vi "SteeringControl.vi"(0 "Position (Counts)":i32, 1 "Roll rate (rad/s)":dbl, 2 "RollRef":dbl, 3 "Limit":i8, 4 "P gain":dbl, 5 "I gain":dbl, 6 "error in (no error)":errorcluster, 7 "D gain":dbl, 8 "Time step (s)":dbl, 10 "Roll":dbl) -> (20 "error out":errorcluster, 21 "PWM Out":dbl)   [LabVIEW 2019]
uses:
  <vilib>/myRIO/Instrument Drivers/Onboard IO/PWM/typedefs/PWM Reference.ctl
  <vilib>/myRIO/Common/Instrument Driver Framework/Utilities/typedefs/myRIO Generic Hardware Reference.ctl
  <vilib>/myRIO/Common/Instrument Driver Framework/Utilities/typedefs/Hardware Version Enum.ctl
  <vilib>/myRIO/Common/Instrument Driver Framework/Utilities/typedefs/myRIO v1.0 Reference.ctl
  <vilib>/myRIO/Common/Instrument Driver Framework/Utilities/typedefs/Generic FPGA Reference.ctl
  <vilib>/myRIO/Common/Instrument Driver Framework/myRIO v1.0/PWM/typedefs/PWM Channels Enum.ctl
  <vilib>/myRIO/Instrument Drivers/Onboard IO/PWM/typedefs/PWM Configuration.ctl
  <vilib>/userDefined/High Color/nirio_resource_hc.ctl
  <vilib>/myRIO/Common/Instrument Driver Framework/Utilities/vis/Is FPGA Ref Available.vi
  <vilib>/myRIO/Common/Instrument Driver Framework/myRIO v1.0/PWM/vis/myRIO v1.1 Open PWM.vi
  <vilib>/myRIO/Instrument Drivers/Onboard IO/PWM/vis/Set Duty Cycle and Frequency.vi
  <vilib>/myRIO/Common/Instrument Driver Framework/Utilities/vis/Validate Channels.vi
  <vilib>/myRIO/Common/Instrument Driver Framework/myRIO v1.0/PWM/vis/myRIO v1.0 Reserve PWM.vi
  <vilib>/myRIO/Common/Instrument Driver Framework/myRIO v1.0/PWM/vis/myRIO v1.0 Build MUX Configuration PWM.vi
  <vilib>/myRIO/Common/Instrument Driver Framework/myRIO v1.0/Resource Manager/vis/myRIO v1.0 Reserve Channel List.vi
  <vilib>/myRIO/Common/Instrument Driver Framework/myRIO v1.0/Resource Manager/vis/myRIO v1.0 Create Configuration List.vi
  <vilib>/myRIO/Common/Instrument Driver Framework/myRIO v1.0/Resource Manager/vis/myRIO v1.0 Reserve Channel.vi
  <vilib>/myRIO/Common/Instrument Driver Framework/myRIO v1.0/Resource Manager/vis/myRIO v1.0 Unreserve Channel.vi
  <vilib>/myRIO/Common/Instrument Driver Framework/myRIO v1.0/Resource Manager/vis/myRIO v1.0 Build Mutex Name.vi
  <vilib>/Utility/VariantDataType/GetNumericInfo.vi
  <vilib>/Utility/error.llb/Error Cluster From Error Code.vi
  <vilib>/myRIO/Common/Instrument Driver Framework/myRIO v1.0/myRIO v1.1 Open.vi
  <vilib>/myRIO/Common/Instrument Driver Framework/Utilities/vis/IO Manager.vi
  <vilib>/myRIO/Common/Instrument Driver Framework/Utilities/vis/Configuration Manager.vi
  <vilib>/myRIO/Common/Instrument Driver Framework/myRIO v1.0/Resource Manager/vis/myRIO v1.0 Configure IO.vi
  <vilib>/myRIO/Common/Instrument Driver Framework/myRIO v1.0/myRIO v1.0 Close.vi
  <vilib>/myRIO/Common/Instrument Driver Framework/myRIO v1.0/PWM/vis/myRIO v1.0 Write PWM.vi
  <vilib>/myRIO/Express VI/Onboard IO/PWM/PWM Express VI.xnode
  <vilib>/myRIO/Instrument Drivers/Onboard IO/PWM/vis/myRIO PWM Open.xnode
  <vilib>/myRIO/Instrument Drivers/Onboard IO/PWM/PWM.lvlib
  libbalancing2.dll
panel:
  out "PWM from C out":dbl
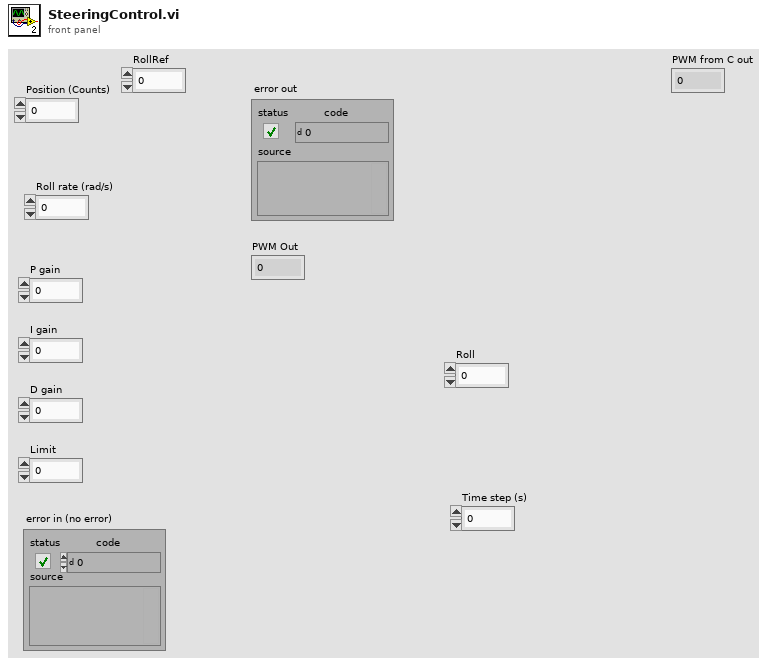
[diagram p1: front panel]
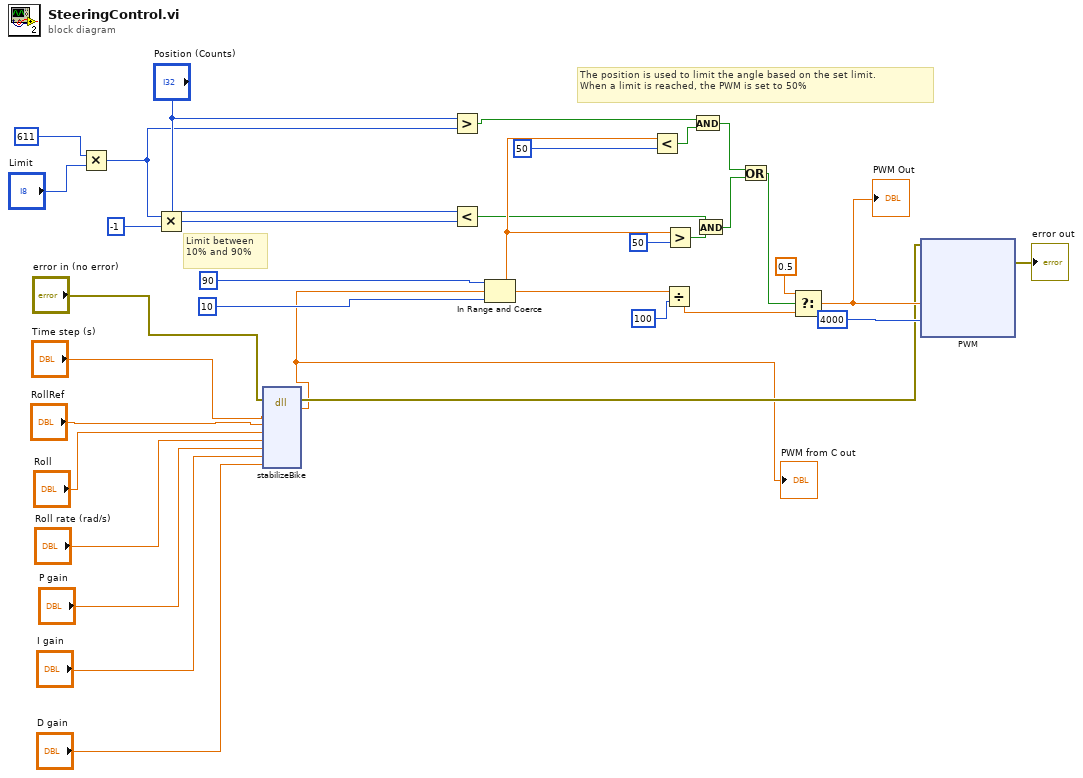
[diagram p0: block diagram]
diagram:
  # "Limit between\n10% and 90%"
  # "The position is used to limit the angle based on the set limit.\nWhen a limit is reached, the PWM is set to 50%"
  n1 = Multiply(x=611, y="Limit") -> (x*y=w13:i32)
  n2 = Multiply(x=w13, y=-1) -> (x*y=w15:i32)
  n3 = dll-call lib="libbalancing2.*" fn="stabilizeBike"(error in="error in (no error)", "timestep"="Time step (s)", "referenceroll"="RollRef", "roll"="Roll", "rollrate"="Roll rate (rad/s)", "kp"="P gain", "ki"="I gain", "kd"="D gain") -> (error out=w2:errorcluster, "return type"=w1:dbl)  [unwired: 9 in, 1 out]
  "PWM from C out" <- w1
  n4 = Greater?(x="Position (Counts)", y=w13) -> (0:w34:bool)
  n5 = Less?(x="Position (Counts)", y=w15) -> (x < y?=w22:bool)
  n6 = In Range and Coerce(upper limit=90, x=w1, lower limit=10) -> (coerced(x)=w26:dbl)  [unwired: 1 out]
  n7 = Less?(x=w26, y=50) -> (x < y?=w25:bool)
  n8 = Divide(x=w26, y=100) -> (x/y=w31:dbl)
  n9 = Greater?(x=w26, y=50) -> (0:w23:bool)
  n10 = And(x=w34, y=w25) -> (x .and. y?=w28:bool)
  n11 = And(x=w22, y=w23) -> (x .and. y?=w29:bool)
  n12 = Or(x=w28, y=w29) -> (x .or. y?=w30:bool)
  n13 = Select(t=0.5, s=w30, f=w31) -> (s? t:f=w11:dbl)
  "PWM Out" <- w11
  n14 = xnode "PWM"("Duty Cycle"=w11, "Frequency [Hz]"=4000, "error in (no error)"=w2) -> ("error out"=→"error out":errorcluster)
